vi "17-FindVy.vi"(10 "Vx":T1(array[cluster]), 11 "Target":T2) -> (2 "Max Y":i32, 3 "N Solutions":i32)   [LabVIEW 2019, in "17.lvlib"]
uses:
  6da09b54-7182-4690-9fd5-0358925057ba.vi
  <vilib>/Analysis/1siggen.llb/Ramp Pattern by Delta.vi
  17.lvlib
  <vilib>/Analysis/NI_AALBase.lvlib
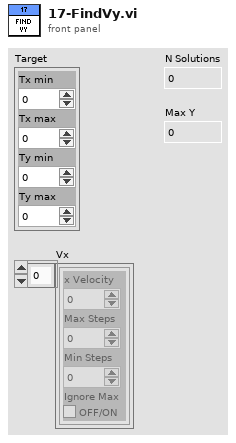
[diagram p1: front panel]
types:
  T1 = cluster{"x Velocity":i32, "Max Steps":i32, "Min Steps":i32, "Ignore Max":bool}[]
  T2 = cluster{"Tx min":i32, "Tx max":i32, "Ty min":i32, "Ty max":i32}
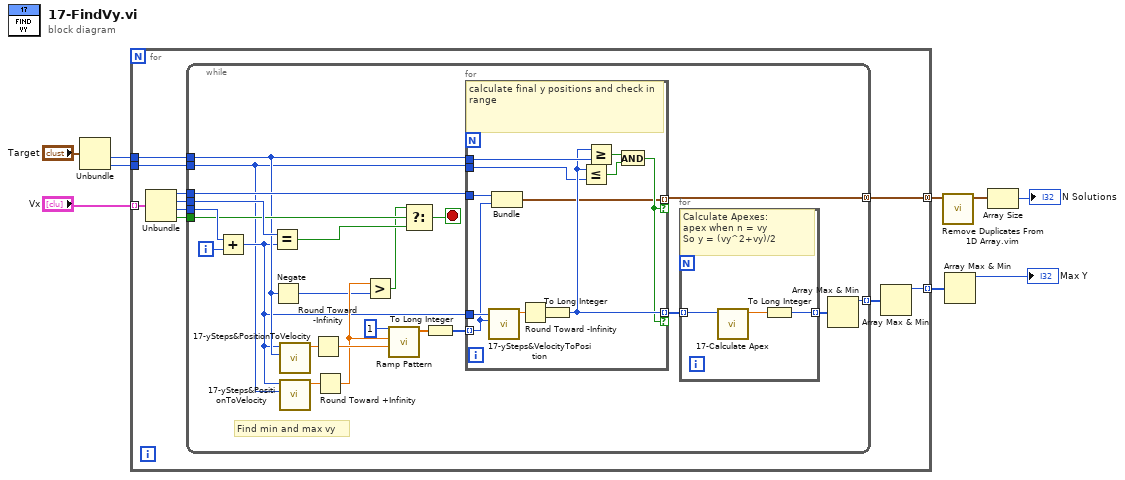
[diagram p0: block diagram]
diagram:
  n1 = Unbundle("Target") -> ("Ty min"=w7:i32, "Ty max"=w8:i32)  [unwired: 2 out]
  n2 = for {
    tunnel: w7 -> [w19]
    tunnel: w8 -> [w18]
    tunnel: [w16] -> w3 mode=indexing
    tunnel: [w15] -> w1 mode=concatenating
    tunnel: "Vx" -> [w13] mode=indexing
    n3 = Unbundle(w13) -> ("x Velocity"=w10:i32, "Max Steps"=w11:i32, "Min Steps"=w12:i32, "Ignore Max"=w14:bool)
    n4 = while {
      tunnel: w19 -> [w24]
      tunnel: w18 -> [w21]
      tunnel: [w38] -> w17 mode=indexing
      tunnel: w10 -> [w36]
      tunnel: [w35] -> w15 mode=concatenating
      tunnel: w11 -> [w29]
      tunnel: w14 -> [w27]
      tunnel: w12 -> [w32]
      i -> [w23]
      stop <- w28 stop-if-true
      # "Find min and max vy"
      n5 = Add(x=w32, y=w23) -> (x+y=w22:i32)
      n6 = Equal?(x=w29, y=w22) -> (x = y?=w26:bool)
      n7 = Negate(x=w24) -> (-x=w30:i32)
      n8 = call "17-ySteps&PositionToVelocity.vi"("y"=w24, "n"=w22) -> ("vy"=w40:dbl)  [unwired: 9 in]
      n9 = call "17-ySteps&PositionToVelocity.vi"("y"=w21, "n"=w22) -> ("vy"=w20:dbl)  [unwired: 9 in]
      n10 = Round Toward -Infinity(1:w40) -> (0:w34:dbl)
      n11 = Round Toward +Infinity(x=w20) -> (ceil(x): smallest int >= x=w31:dbl)
      n12 = Greater?(x=w31, y=w30) -> (0:w25:bool)
      n13 = call-poly <vilib>:"Ramp Pattern.vi"("start"=w34, "end"=w31, "delta"=1 ("Tx max")) -> ("Ramp Pattern"=w42:dbl[])  [unwired: 6 in, 2 out]
      n14 = Select(t=w25, s=w27, f=w26) -> (s? t:f=w28:bool)
      n15 = To Long Integer(number=w42) -> (32bit integer=w41:i32[])
      n16 = for {
        tunnel: w41 -> [w50] mode=indexing
        tunnel: w22 -> [w57]
        tunnel: [w54] -> w37 mode=indexing if=w49
        tunnel: w24 -> [w55]
        tunnel: w21 -> [w53]
        tunnel: [w48] -> w35 mode=indexing if=w49
        tunnel: w36 -> [w47]
        # "calculate final y positions and check in range"
        n17 = call "17-ySteps&VelocityToPosition.vi"("vy"=w50, "n"=w57) -> ("y"=w56:dbl)  [unwired: 9 in]
        n18 = Bundle("x Velocity"=w47, w50) -> (w48:cluster{"x Velocity":i32, i32})  [unwired: 1 in]
        n19 = Round Toward -Infinity(1:w56) -> (0:w46:dbl)
        n20 = To Long Integer(number=w46) -> (32bit integer=w54:i32)
        n21 = Less Or Equal?(x=w54, y=w53) -> (x <= y?=w51:bool)
        n22 = Greater Or Equal?(x=w54, y=w55) -> (x >= y?=w52:bool)
        n23 = And(x=w52, y=w51) -> (x .and. y?=w49:bool)
      }
      n24 = for {
        tunnel: w37 -> [w43] mode=indexing
        tunnel: [w44] -> w39 mode=indexing
        # "Calculate Apexes:\napex when n = vy\nSo y = (vy^2+vy)/2"
        n25 = call "17-Calculate Apex.vi"("vy"=w43) -> ("y"=w45:dbl)  [unwired: 10 in]
        n26 = To Long Integer(number=w45) -> (32bit integer=w44:i32)
      }
      n27 = Array Max & Min(array=w39) -> (max value=w38:i32)  [unwired: 3 out]
    }
    n28 = Array Max & Min(array=w17) -> (max value=w16:i32)  [unwired: 3 out]
  }
  n29 = call "Remove Duplicates From 1D Array.vim"("array"=w1) -> ("array with duplicates removed"=w2:cluster{"x Velocity":i32, i32}[])  [unwired: 10 in]
  n30 = Array Max & Min(array=w3) -> (max value=→"Max Y":i32)  [unwired: 3 out]
  n31 = Array Size(array=w2) -> (size(s)=→"N Solutions":i32)
